vi "Initialize Device Core.vi"(8 "error in (no error)":errorcluster, 9 "Reset (F)":bool, 10 "Resource Name":string, 11 "CS++Nanotec in":refnum<class "CS++Nanotec.lvclass">) -> (0 "error out":errorcluster, 3 "CS++Nanotec out":refnum<class "CS++Nanotec.lvclass">)   [LabVIEW 2015, in "CS++Nanotec.lvlib" / "CS++Nanotec.lvclass"]
doc: "Initialize device driver."
uses:
  CS++Nanotec.lvclass
  CS++Nanotec.lvclass/CS++Nanotec.ctl
  CSPP_DeviceBase/CS++Motor/CS++Motor.lvclass
  instr.lib/NanotecSMCPD/NanotecSMCPDDriver.lvlib
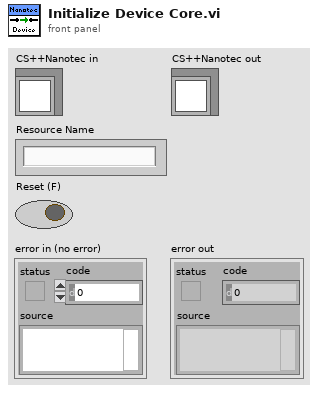
[diagram p1: front panel]
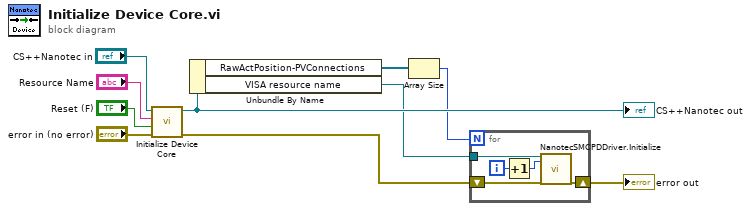
[diagram p0: block diagram]
diagram:
  n1 = call-parent "Initialize Device Core.vi"("error in (no error)"="error in (no error)", "Reset (F)"="Reset (F)", "Resource Name"="Resource Name", "CS++Motor in"="CS++Nanotec in") -> ("error out"=w3:errorcluster, "CS++Motor out"=w6:refnum<class "CS++Nanotec.lvclass">)  [unwired: 6 in]
  "CS++Nanotec out" <- w6
  n2 = Unbundle By Name(w6) -> ("RawActPosition-PVConnections"=w5:refnum<class "PVConnection.lvclass">[], "VISA resource name"=w4:refnum<visa-resource-name>)
  n3 = Array Size(array=w5) -> (size(s)=w1:i32)
  n4 = for {
    N: w1 -> [_]
    tunnel: w4 -> [w15]
    shift-right: [w13] -> w2
    shift-left: w3 -> [w14]
    i -> [w12]
    n5 = Increment(x=w12) -> (x+1=w11:i32)
    n6 = call "NanotecSMCPDDriver.Initialize.vi"("VISA resource name"=w15, "contollerID"=w11, "error in (no error)"=w14) -> ("error out"=w13:errorcluster)  [unwired: 14 in, 2 out]
  }
  "error out" <- w2
